vi "LSR Make Transmission.vi"(8 "error in (no error)":errorcluster, 11 "Data String":string) -> (0 "error out":errorcluster, 3 "Transmission":string[](array[string]))   [LabVIEW 2015, in "LSR Transmission.lvlib"]
doc: "This VI splits up an incoming string (which is flattened object data) to packets of a set length. it then creates stuffed COBS packets and adds a header packet which contains the number of packets in the transmission not including the header."
uses:
  LSR Transmission.lvlib
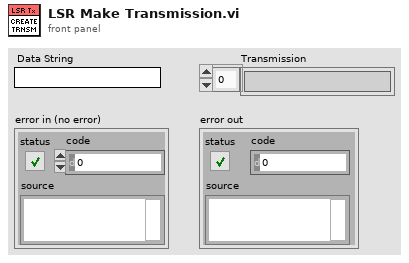
[diagram p1: front panel]
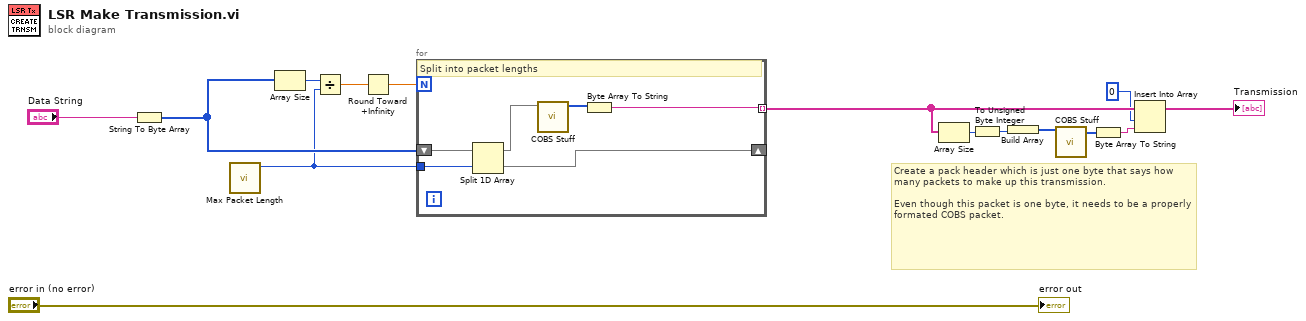
[diagram p0: block diagram]
diagram:
  # "Create a pack header which is just one byte that says how many packets to make up this transmission.\n\nEven though this packet is one byte, it needs to be a properly formated COBS packet."
  n1 = String To Byte Array(string="Data String") -> (unsigned byte array=w8:u8[])
  n2 = call "Max Packet Length.vi"() -> ("Max Packet Length"=w5:i32)  [unwired: 11 in]
  n3 = Array Size(array=w8) -> (size(s)=w7:i32)
  n4 = Divide(x=w7, y=w5) -> (x/y=w13:dbl)
  n5 = Round Toward +Infinity(x=w13) -> (ceil(x): smallest int >= x=w14:dbl)
  n6 = for {
    N: w14 -> [_]
    shift-right: [w19] -> _
    shift-left: w8 -> [w20]
    tunnel: w5 -> [w21]
    tunnel: [w16] -> w15 mode=indexing
    # "Split into packet lengths"
    n7 = Split 1D Array(array=w20, index=w21) -> (first subarray=w18:u8[], second subarray=w19:u8[])
    n8 = call "COBS Stuff.vi"("Raw Array in"=w18) -> ("Stuffed Array out"=w17:u8[])  [unwired: 9 in, 1 out]
    n9 = Byte Array To String(unsigned byte array=w17) -> (string=w16:string)
  }
  n10 = Array Size(array=w15) -> (size(s)=w12:i32)
  n11 = To Unsigned Byte Integer(number=w12) -> (unsigned 8bit integer=w4:u8)
  n12 = Build Array(w4) -> (w3:u8[])
  n13 = call "COBS Stuff.vi"("Raw Array in"=w3) -> ("Stuffed Array out"=w2:u8[])  [unwired: 9 in, 1 out]
  n14 = Byte Array To String(unsigned byte array=w2) -> (string=w1:string)
  n15 = Insert Into Array(array=w15, index=0, new element=w1) -> (→"Transmission":string[])
  "error out" <- "error in (no error)"
